vi "Initialize Galil.vi"(0 "Galil.IGalil":refnum<k7>, 1 "Initial Encoder Counts":string="0" caption="Enter number in encoder counts, 0 is middle, -650000 fully entended; 650000 fully retracted", 12 "Disabled?":bool) -> (4 "reference out 3":refnum<k7>, 5 "address":string="192.168.1.10", 6 "error out 3":errorcluster, 9 "timeout_ms":i32=500, 14 "Output String":string, 15 "Error Query Connection":errorcluster)   [LabVIEW 2011]
panel:
  out "error out 2":errorcluster
  out "addresses":variant
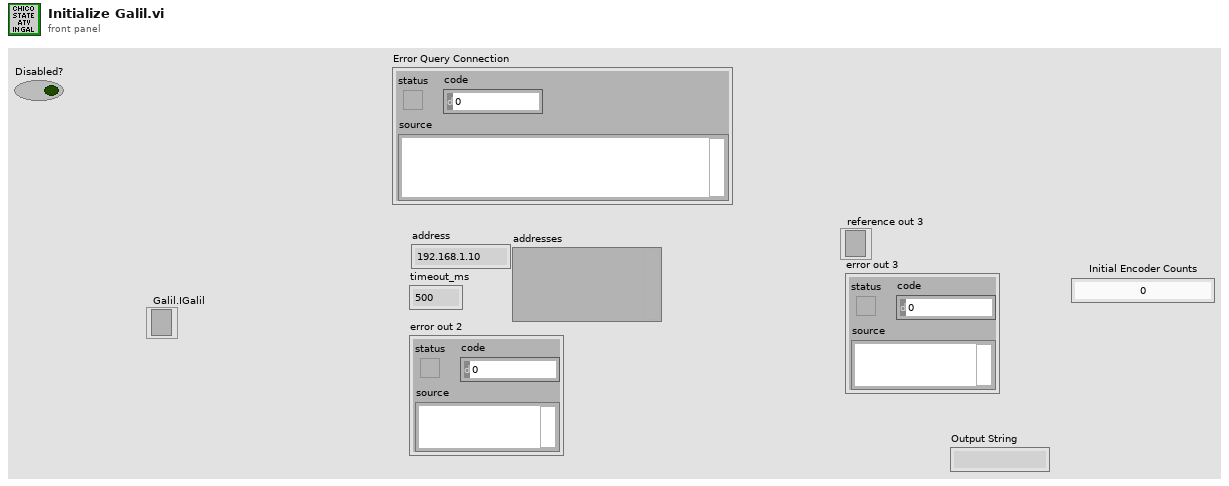
[diagram p1: front panel]
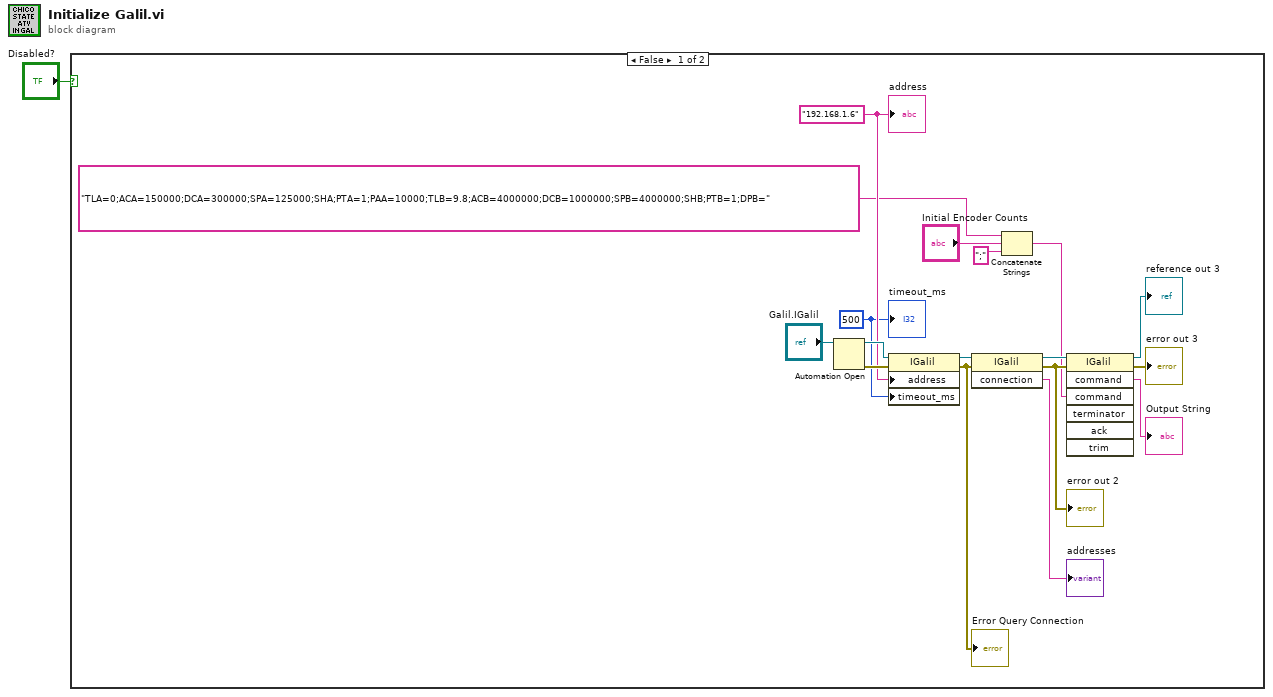
[diagram p0: block diagram]
diagram:
  n1 = case shown="False" "Disabled?" {
    frame False {
      w6 = 500 ("timeout_ms")
      w7 = "192.168.1.6" ("address")
      n2 = Automation Open(Automation Refnum="Galil.IGalil") -> (Automation Refnum=w15:refnum<k7>, error out=w14:errorcluster)  [unwired: 3 in]
      n3 = property class="IGalil"(reference=w15, error in=w14, "address"=w7, "timeout_ms"=w6) -> (reference out=w11:refnum<k7>, error out=w12:errorcluster)
      "Error Query Connection" <- w12
      n4 = invoke class="IGalil" method="connection"(reference=w11, error in=w12) -> (reference out=w8:refnum<k7>, error out=w9:errorcluster, "connection"=→"addresses":string)  [unwired: 1 in]
      "error out 2" <- w9
      n5 = Concatenate Strings("TLA=0;ACA=150000;DCA=300000;SPA=125000;SHA;PTA=1;PAA=10000;TLB=9.8;ACB=4000000;DCB=1000000;SPB=4000000;SHB;PTB=1;DPB=" ("Command Input"), "Initial Encoder Counts", ";" ("string")) -> (w2:string)
      n6 = invoke class="IGalil" method="command"(reference=w8, error in=w9, "command"=w2) -> (reference out=→"reference out 3":refnum<k7>, error out=→"error out 3":errorcluster, "command"=→"Output String":string)  [unwired: 4 in, 4 out]
      "address" <- w7
      "timeout_ms" <- w6
    }
    frame True {
    }
  }
